vi "Ballard - 1553 - Load Database.vi"(8 "error in (no error)":errorcluster, 11 "Node Ptr":u64 format="%.0x") -> (0 "error out":errorcluster)   [LabVIEW 2020, in "Ballard 1553 System Explorer.lvlib"]
uses:
  Ballard 1553 System Explorer.lvlib
panel:
  in  "Tag":string
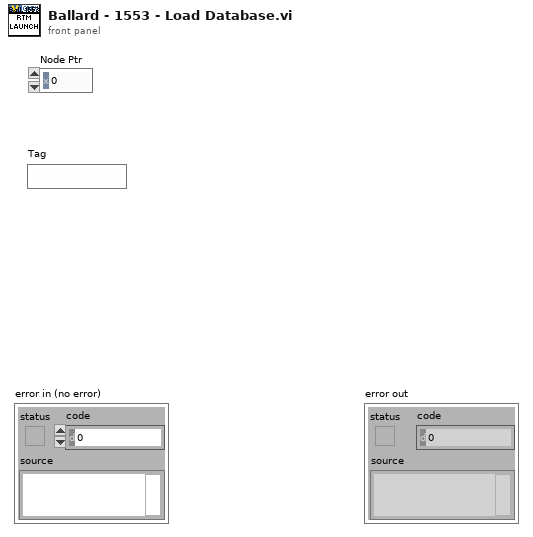
[diagram p1: front panel]
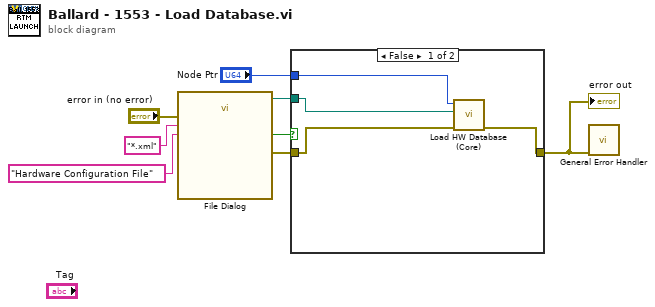
[diagram p0: block diagram]
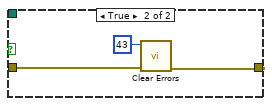
[diagram p2: hidden frame]
diagram:
  n1 = call "File Dialog"("error in"="error in (no error)", "pattern (all files)"="*.xml", "pattern label"="Hardware Configuration File") -> ("selected path"=w1:path, "cancelled"=w4:bool, "error out"=w3:errorcluster)  [unwired: 9 in, 1 out]
  n2 = case shown="False" w4 {
    tunnel: [w12 w13] -> w8
    tunnel: w3 -> [w11 w14]
    tunnel: "Node Ptr" -> [w10 _]
    tunnel: w1 -> [w9 _]
    frame False {
      n3 = call "Load HW Database (Core).vi"("error in"=w11, "hw db path in"=w9, "Node Ptr"=w10) -> ("error out"=w12:errorcluster)  [unwired: 8 in]
    }
    frame True {
      n4 = call <vilib>:"Clear Errors.vi"("error in (no error)"=w14, "specific error code to clear (0: all)"=43) -> ("error out"=w13:errorcluster)  [unwired: 4 in, 1 out]
    }
  }
  "error out" <- w8
  n5 = call <vilib>:"General Error Handler.vi"("error in (no error)"=w8) -> ()  [unwired: 10 in, 5 out]
